vi "BK1900 Driver.vi"(0 "VISA Refnum in":refnum<visa-resource-name>, 1 "data bits (8)":u16, 2 "parity (0:none)":enum16{"None", "Odd", "Even", "Mark", "Space"}(ring), 3 "INPUT CURRENT":dbl, 4 "stop bits (10: 1 bit)":u16, 6 "baud rate":u32, 7 "flow control (0:none)":u16, 8 "Message Based Settings:Send End Enable 2":bool, 9 "Termination Character":u8, 10 "INPUT VOLTAGE":dbl, 11 "Serial Settings:Serial End Mode for Writes":u16, 13 "Message Based Settings:Send End Enable":bool) -> (14 "Numeric 2":dbl, 15 "Numeric":dbl, 19 "error out":errorcluster)   [LabVIEW 2025]
uses:
  <vilib>/Instr/_visa.llb/VISA Configure Serial Port (Instr).vi
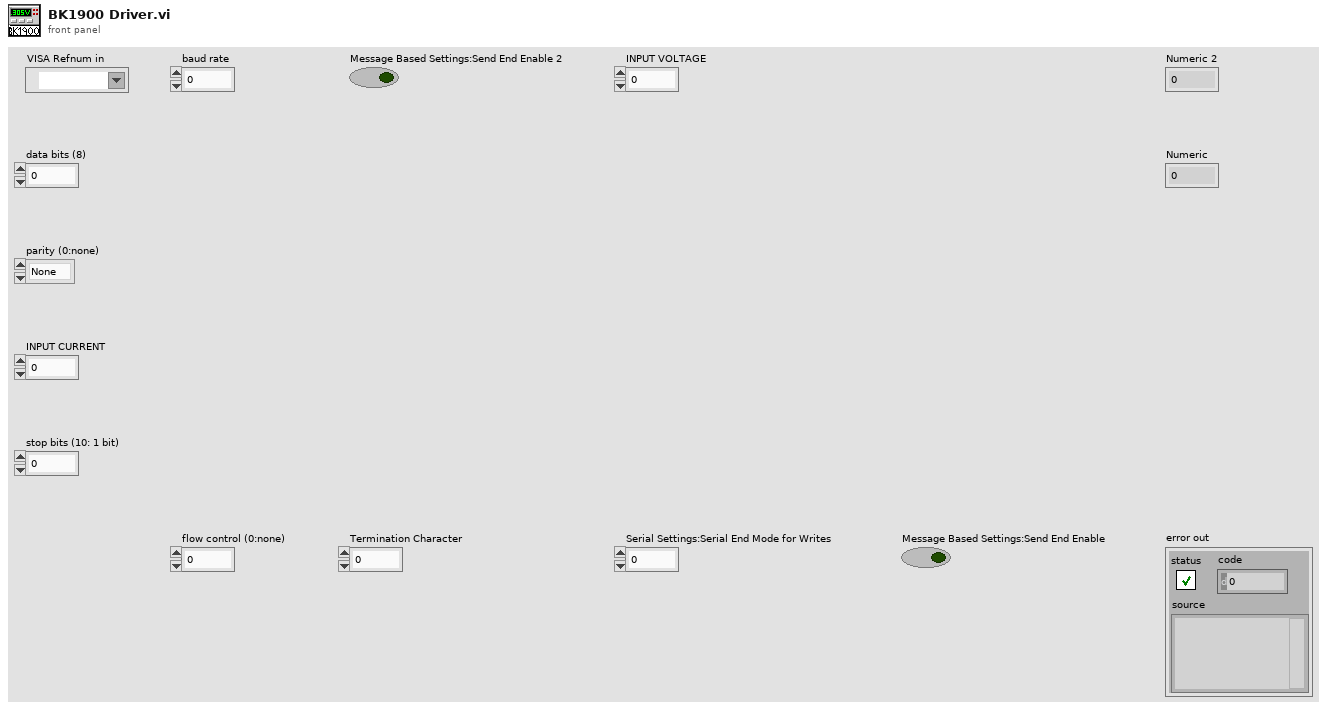
[diagram p1: front panel]
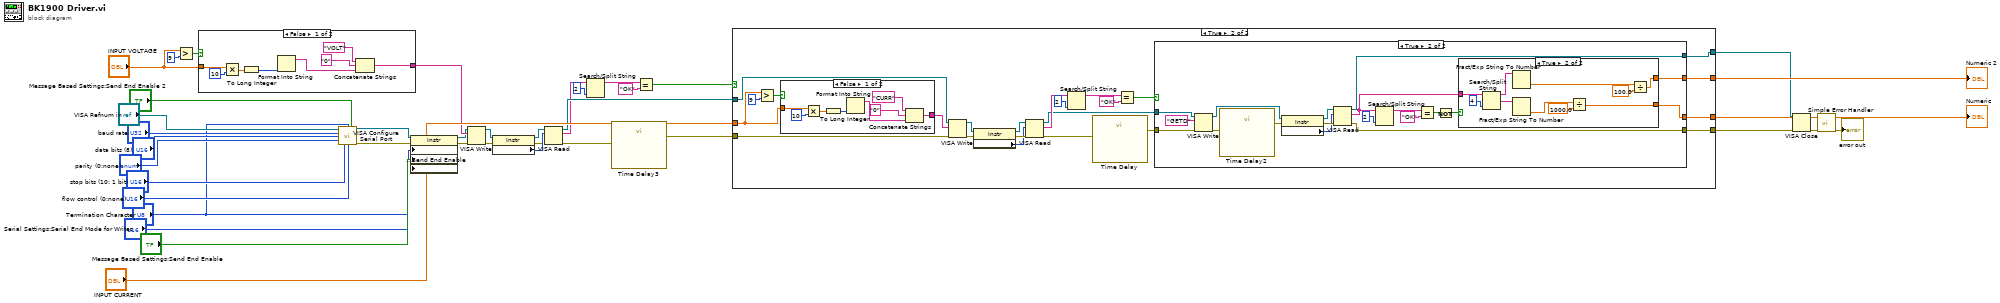
[diagram p0: block diagram]
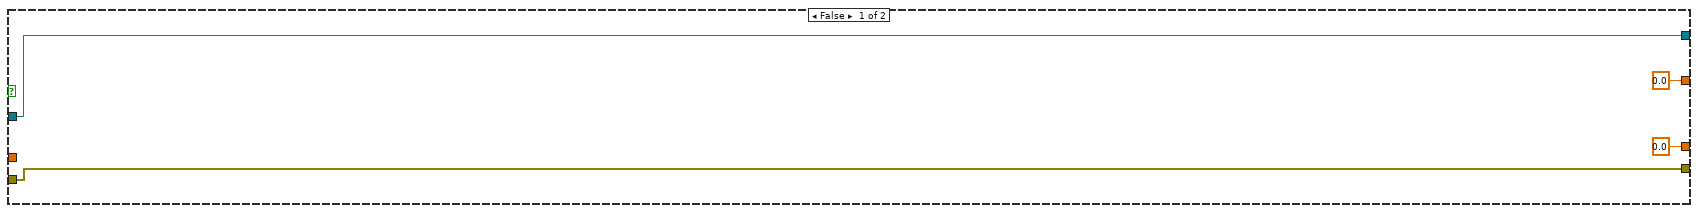
[diagram p2: hidden frame]
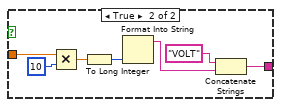
[diagram p3: hidden frame]
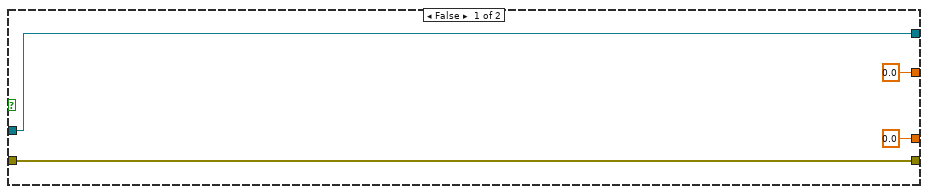
[diagram p4: hidden frame]
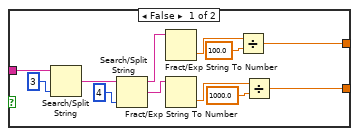
[diagram p5: hidden frame]
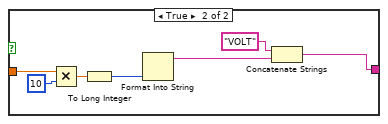
[diagram p6: hidden frame]
diagram:
  n1 = Greater?(x="INPUT VOLTAGE", y=u32 9) -> (0:w19:bool)
  n2 = case shown="False" w19 {
    tunnel: [w43 w52] -> w21
    tunnel: "INPUT VOLTAGE" -> [w42 w50]
    frame False {
      n3 = Multiply(x=w42, y=u32 10) -> (x*y=w40:dbl)
      n4 = To Long Integer(number=w40) -> (32bit integer=w39:i32)
      n5 = Format Into String(w39) -> (resulting string=w44:string)  [unwired: 3 in, 1 out]
      n6 = Concatenate Strings("VOLT" ("string"), "0" ("string"), w44) -> (w43:string)
    }
    frame True {
      n7 = Multiply(x=w50, y=u32 10) -> (x*y=w48:dbl)
      n8 = To Long Integer(number=w48) -> (32bit integer=w47:i32)
      n9 = Format Into String(w47) -> (resulting string=w51:string)  [unwired: 3 in, 1 out]
      n10 = Concatenate Strings("VOLT" ("string"), w51) -> (w52:string)
    }
  }
  n11 = call-poly "VISA Configure Serial Port"("VISA resource name"="VISA Refnum in", "termination char\n(0xA = '\\n' = LF)"="Termination Character", "Enable Termination\nChar (T)"="Message Based Settings:Send End Enable 2", "baud rate (9600)"="baud rate", "data bits (8)"="data bits (8)", "parity (0:none)"="parity (0:none)", "stop bits (10: 1 bit)"="stop bits (10: 1 bit)", "flow control (0:none)"="flow control (0:none)") -> ("VISA resource name out"=w11:refnum<visa-resource-name>, "error out"=w12:errorcluster)  [unwired: 2 in, 4 out]
  n12 = property class="Instr"(reference=w11, error in=w12, "Serial Settings:End Mode for Writes"="Serial Settings:Serial End Mode for Writes", "Message Based Settings:Send End Enable"="Message Based Settings:Send End Enable", "Message Based Settings:Termination Character"="Termination Character") -> (reference out=w15:refnum<visa-resource-name>, error out=w16:errorcluster)
  n13 = VISA Write(VISA resource name=w15, write buffer=w21, error in (no error)=w16) -> (VISA resource name out=w25:refnum<visa-resource-name>, error out=w26:errorcluster)  [unwired: 1 out]
  n14 = property class="Instr"(reference=w25, error in=w26) -> (reference out=w23:refnum<visa-resource-name>, error out=w22:errorcluster, "Serial Settings:Number of Bytes at Serial Port"=w24:u32)
  n15 = VISA Read(VISA resource name=w23, byte count=w24, error in (no error)=w22) -> (VISA resource name out=w31:refnum<visa-resource-name>, read buffer=w27:string, error out=w33:errorcluster)  [unwired: 1 out]
  n16 = Search/Split String(string=w27, offset (0)=2) -> (substring before match=w29:string)  [unwired: 1 in, 2 out]
  n17 = call "Time Delay3"("error in (no error)"=w33) -> ("error out"=w34:errorcluster)  [unwired: 10 in]
  n18 = Equal?(x=w29, y="OK") -> (x = y?=w32:bool)
  n19 = case shown="True" w32 {
    tunnel: w31 -> [w57 w80]
    tunnel: w34 -> [w56 w79]
    tunnel: [w57 w68] -> w17
    tunnel: [w56 w67] -> w18
    tunnel: [0.0 w60] -> w36
    tunnel: [0.0 w59] -> w37
    tunnel: "INPUT CURRENT" -> [_ w58]
    frame False {
    }
    frame True {
      n20 = Greater?(x=w58, y=u32 9) -> (0:w63:bool)
      n21 = case shown="False" w63 {
        tunnel: [w85 w94] -> w61
        tunnel: w58 -> [w84 w92]
        frame False {
          n22 = Multiply(x=w84, y=u32 10) -> (x*y=w82:dbl)
          n23 = To Long Integer(number=w82) -> (32bit integer=w81:i32)
          n24 = Format Into String(w81) -> (resulting string=w86:string)  [unwired: 3 in, 1 out]
          n25 = Concatenate Strings("CURR" ("string"), "0" ("string"), w86) -> (w85:string)
        }
        frame True {
          n26 = Multiply(x=w92, y=u32 10) -> (x*y=w90:dbl)
          n27 = To Long Integer(number=w90) -> (32bit integer=w89:i32)
          n28 = Format Into String(w89) -> (resulting string=w93:string)  [unwired: 3 in, 1 out]
          n29 = Concatenate Strings("VOLT" ("string"), w93) -> (w94:string)
        }
      }
      n30 = VISA Write(VISA resource name=w80, write buffer=w61, error in (no error)=w79) -> (VISA resource name out=w78:refnum<visa-resource-name>, error out=w77:errorcluster)  [unwired: 1 out]
      n31 = property class="Instr"(reference=w78, error in=w77) -> (reference out=w76:refnum<visa-resource-name>, error out=w75:errorcluster, "Serial Settings:Number of Bytes at Serial Port"=w74:u32)
      n32 = VISA Read(VISA resource name=w76, byte count=w74, error in (no error)=w75) -> (VISA resource name out=w64:refnum<visa-resource-name>, read buffer=w71:string, error out=w72:errorcluster)  [unwired: 1 out]
      n33 = Search/Split String(string=w71, offset (0)=2) -> (substring before match=w69:string)  [unwired: 1 in, 2 out]
      n34 = call "Time Delay"("error in (no error)"=w72) -> ("error out"=w65:errorcluster)  [unwired: 10 in]
      n35 = Equal?(x=w69, y="OK") -> (x = y?=w66:bool)
      n36 = case shown="True" w66 {
        tunnel: [w99 w115] -> w68
        tunnel: [w98 w114] -> w67
        tunnel: w64 -> [w99 w113]
        tunnel: w65 -> [w98 w112]
        tunnel: [0.0 w101] -> w60
        tunnel: [0.0 w100] -> w59
        frame False {
        }
        frame True {
          n37 = VISA Write(VISA resource name=w113, write buffer="GETD", error in (no error)=w112) -> (VISA resource name out=w118:refnum<visa-resource-name>, error out=w109:errorcluster)  [unwired: 1 out]
          n38 = call "Time Delay2"("error in (no error)"=w109) -> ("error out"=w108:errorcluster)  [unwired: 10 in]
          n39 = property class="Instr"(reference=w118, error in=w108) -> (reference out=w117:refnum<visa-resource-name>, error out=w116:errorcluster, "Serial Settings:Number of Bytes at Serial Port"=w110:u32)
          n40 = VISA Read(VISA resource name=w117, byte count=w110, error in (no error)=w116) -> (VISA resource name out=w115:refnum<visa-resource-name>, read buffer=w102:string, error out=w114:errorcluster)  [unwired: 1 out]
          n41 = Search/Split String(string=w102, offset (0)=2) -> (substring before match=w106:string)  [unwired: 1 in, 2 out]
          n42 = Equal?(x=w106, y="OK") -> (x = y?=w104:bool)
          n43 = Not(x=w104) -> (.not. x?=w103:bool)
          n44 = case shown="True" w103 {
            tunnel: w102 -> [w125 w134]
            tunnel: [w124 w135] -> w101
            tunnel: [w123 w136] -> w100
            frame False {
              n45 = Search/Split String(string=w125, offset (0)=3) -> (match + rest of string=w120:string)  [unwired: 1 in, 2 out]
              n46 = Search/Split String(string=w120, offset (0)=4) -> (substring before match=w119:string, match + rest of string=w121:string)  [unwired: 1 in, 1 out]
              n47 = Fract/Exp String To Number(string=w119) -> (number=w129:dbl)  [unwired: 3 in, 1 out]
              n48 = Fract/Exp String To Number(string=w121) -> (number=w130:dbl)  [unwired: 3 in, 1 out]
              n49 = Divide(x=w129, y=100.0) -> (x/y=w124:dbl)
              n50 = Divide(x=w130, y=1000.0) -> (x/y=w123:dbl)
            }
            frame True {
              n51 = Search/Split String(string=w134, offset (0)=4) -> (substring before match=w132:string, match + rest of string=w131:string)  [unwired: 1 in, 1 out]
              n52 = Fract/Exp String To Number(string=w132) -> (number=w139:dbl)  [unwired: 3 in, 1 out]
              n53 = Fract/Exp String To Number(string=w131) -> (number=w140:dbl)  [unwired: 3 in, 1 out]
              n54 = Divide(x=w140, y=1000.0) -> (x/y=w136:dbl)
              n55 = Divide(x=w139, y=100.0) -> (x/y=w135:dbl)
            }
          }
        }
      }
    }
  }
  "Numeric" <- w37
  "Numeric 2" <- w36
  n56 = VISA Close(VISA resource name=w17, error in (no error)=w18) -> (error out=w8:errorcluster)
  n57 = call <vilib>:"Simple Error Handler.vi"("error in (no error)"=w8) -> ("error out"=→"error out":errorcluster)  [unwired: 1 in, 7 out]
